vi "Capture.vi"(8 "Error":errorcluster, 11 "KNR in":T1) -> (0 "error out":errorcluster, 2 "Image Out":T3(plugin-control), 3 "KNR out":T1)   [LabVIEW 2013]
uses:
  <userlib>/KNR OS 3.0 LabVIEW Toolkit/Type Definition/KNR3 Reference.ctl
  <userlib>/_FPGA Interface Advanced Tools/FPGA Interface Base/FPGA Interface Base.lvclass
  <userlib>/KNR OS 3.0 LabVIEW Toolkit/Type Definition/Resource.ctl
  <vilib>/Platform/TimedLoop/XDataNode/timing_clust.ctl
  <vilib>/Platform/TimedLoop/XDataNode/nitl_modes.ctl
  <vilib>/Platform/TimedLoop/XDataNode/wakeup.ctl
  <vilib>/platform/TimedLoop/XDataNode/XDataNode.xnode
  <vilib>/Platform/TimedLoop/XDataNode/XDNodeRunTimeDep.lvlib
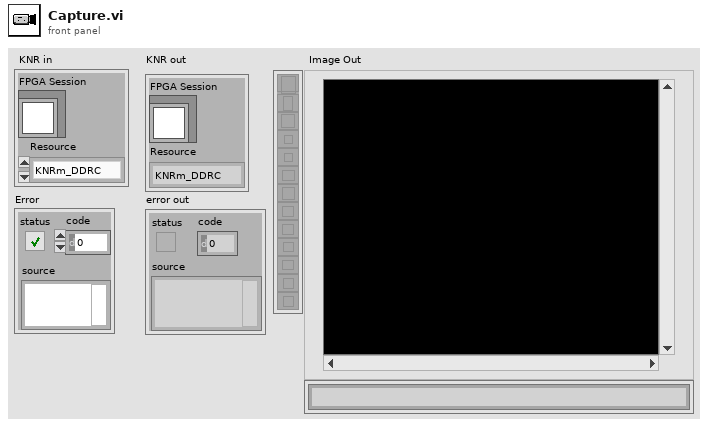
[diagram p1: front panel]
types:
  T1 = typedef "KNR3 Reference.ctl" = cluster{"FPGA Session":refnum<class "FPGA Interface Base.lvclass">, "Resource":T2}
  T2 = typedef "Resource.ctl" = enum16{"KNRm_DDRC", "KNRm_DDDD", "KNRm_DDDR", "KNRm_DDDC", "KNR"}
  T3 = typedef "IMAQ Image.ctl" = refnum<image>
  T4 = typedef "XDNodeRunTimeDep.lvlib/timing_clust.ctl" = cluster{"Expected End [f-1]":u64, "Actual End [f-1]":u64, "Finished Late? [f-1]":bool, "Expected End [i-1]":u64, "Actual End [i-1]":u64, "Finished Late? [i-1]":bool, "Expected Start [i]":u64, "Actual Start [i]":u64, "Expected Start [f]":u64, "Actual Start [f]":u64, "Source Name":string, "Structure Name":string, "Period":i64, "Deadline":i64, "Offset":i64, "Start":i64, "Priority":i32, "Timeout":i32, "Mode":T5, "Wakeup Reason":T6, "Error":errorcluster, "Source Type":string, "Secondary Source Type":string, "Global End Time":u64, "Global Start Time":u64, "Frame Duration":u64, "Iteration Duration":u64, "Assigned CPU":i32, "I/O Scan Engine Mode":u32}
  T5 = typedef "XDNodeRunTimeDep.lvlib/nitl_modes.ctl" = enum32{"No Change", "Process missed periods, maintain original phase", "Discard missed periods, maintain original phase", "Process missed periods, ignore original phase", "Discard missed periods, ignore original phase"}
  T6 = typedef "XDNodeRunTimeDep.lvlib/wakeup.ctl" = enum32{"Normal", "Aborted", "Asynchronous wakeup", "Timing source error", "Timed loop error", "Timeout"}
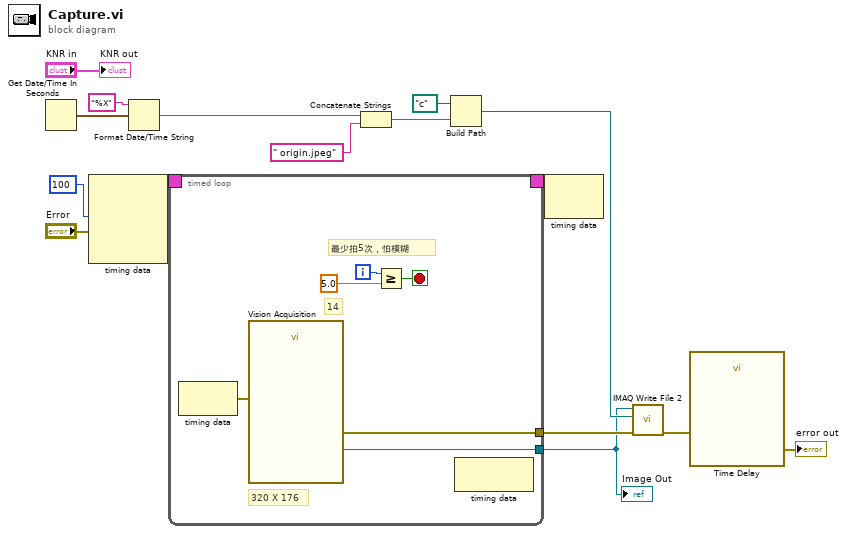
[diagram p0: block diagram]
diagram:
  n1 = Get Date/Time In Seconds() -> (seconds since 1Jan1904=w8:timestamp)
  n2 = node-c288(i64 100 ("Period"), "Error") -> (w16:T4)  [unwired: 2 in]
  n3 = Format Date/Time String(time format string (%c)="%X", seconds (now)=w8) -> (date/time string=w9:string)  [unwired: 1 in]
  n4 = timed-loop {
    timing: w16 -> [_]
    timing-out: [_] -> w15
    tunnel: [w22] -> w2
    tunnel: [w18] -> w7
    i -> [w19]
    stop <- w21 stop-if-true
    # "最少拍5次，怕模糊"
    # "14"
    # "320 X 176"
    n5 = node-c288() -> (w17:errorcluster)  [unwired: 1 in]
    n6 = call "Vision Acquisition"("error in"=w17) -> ("Image Out"=w22:T3, "error out"=w18:errorcluster)  [unwired: 24 in, 1 out]
    n7 = Greater Or Equal?(x=w19, y=5.0) -> (x >= y?=w21:bool)
    n8 = node-c288() -> ()  [unwired: 1 in, 1 out]
  }
  "Image Out" <- w2
  n9 = Concatenate Strings(w9, " origin.jpeg" ("string")) -> (w4:string)
  n10 = Build Path(base path=path "c:/" ("File Path"), name or relative path=w4) -> (appended path=w12:path)
  n11 = node-c288(w15) -> ()  [unwired: 1 out]
  n12 = call-poly "IMAQ Write File 2"("error in (no error)"=w7, "File Path"=w12, "Image"=w2) -> ("error out"=w6:errorcluster)  [unwired: 7 in, 1 out]
  n13 = call "Time Delay"("error in (no error)"=w6) -> ("error out"=→"error out":errorcluster)  [unwired: 10 in]
  "KNR out" <- "KNR in"
